vi "set_origin_by_name.vi"(8 "error in (no error)":errorcluster caption="错误输入（无错误）", 9 "new pos":dbl, 10 "name":string, 11 "MotorSystem 输入":refnum<class "MotorSystem.lvclass">) -> (0 "error out":errorcluster caption="错误输出", 3 "MotorSystem 输出":refnum<class "MotorSystem.lvclass">)   [LabVIEW 2016, in "MotionControl.lvlib" / "MotorSystem.lvclass"]
uses:
  <userlib>/MotionControl/MotorSystem/MotorSystem.lvclass
  <userlib>/MotionControl/MotorSystem/MotorSystem.lvclass/MotorSystem.ctl
  <userlib>/MotionControl/OneMotion/OneMotion.lvclass
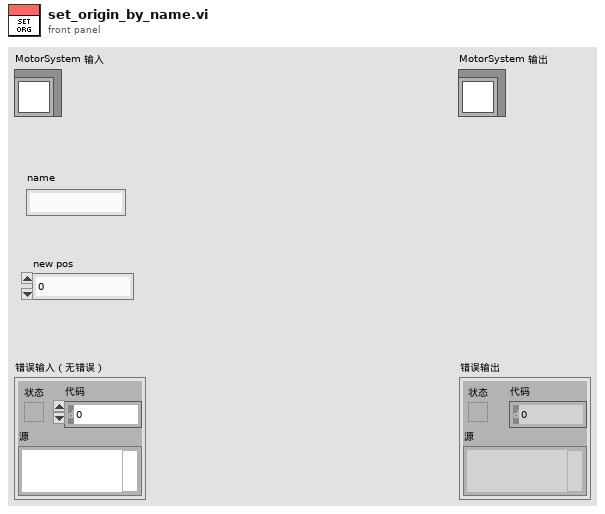
[diagram p1: front panel]
types:
  T1 = typedef "MotionControl.lvlib/MotorSystem.lvclass/MotionCluster.ctl" = cluster{"OneMotion.lvclass":refnum<class "OneMotion.lvclass">, "connected?":bool, "default enabled?":bool, "enabled?":bool}
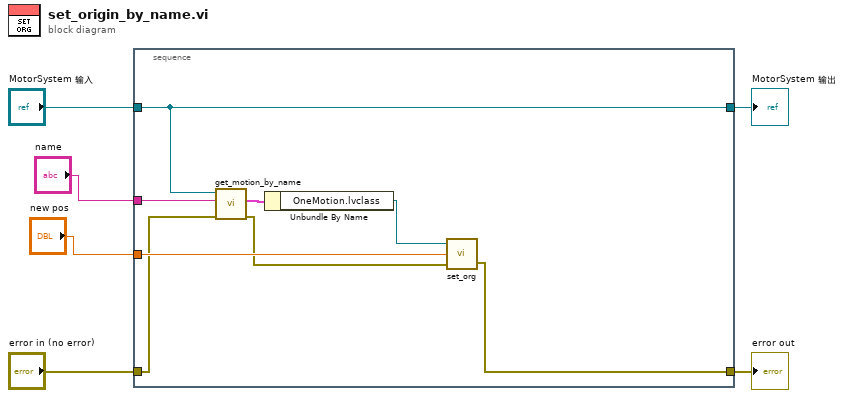
[diagram p0: block diagram]
diagram:
  n1 = stacked-sequence {
    tunnel: [w7] -> w6
    tunnel: [w14] -> w4
    tunnel: "MotorSystem 输入" -> [w14]
    tunnel: "error in (no error)" -> [w9]
    tunnel: "name" -> [w13]
    tunnel: "new pos" -> [w10]
    frame #0 {
      n2 = call <userlib>:"get_motion_by_name.vi"("error in (no error)"=w9, "name"=w13, "MotorSystem in"=w14) -> ("error out"=w8:errorcluster, "motion cluster"=w12:T1)  [unwired: 6 in, 1 out]
      n3 = Unbundle By Name(w12) -> ("OneMotion.lvclass"=w11:refnum<class "OneMotion.lvclass">)
      n4 = call <userlib>:"set_org.vi"("error in (no error)"=w8, "pos"=w10, "OneMotion 输入"=w11) -> ("error out"=w7:errorcluster)  [unwired: 1 out]
    }
  }
  "error out" <- w6
  "MotorSystem 输出" <- w4
